vi "Untitled 4.vi"() -> ()   [LabVIEW 2024]
panel:
  out "logical OR":bool
  out "x != y?":bool[](array[boolean])
  in  "Array 2":i32[](array[numeric])
  in  "Array":i32[](array[numeric])
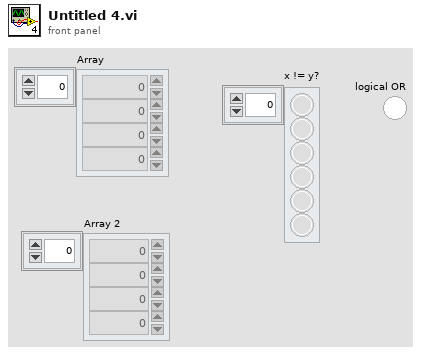
[diagram p1: front panel]
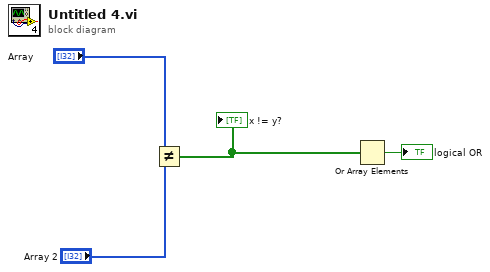
[diagram p0: block diagram]
diagram:
  n1 = Not Equal?(x="Array", y="Array 2") -> (x != y?=w2:bool[])
  "x != y?" <- w2
  n2 = Or Array Elements(Boolean array=w2) -> (logical OR=→"logical OR":bool)
